vi "Board Power Control.vi"(8 "error in (no error)":errorcluster, 9 "VBUS":bool, 10 "Power-On":bool, 11 "CT Common Tests":refnum<class "CT Common Tests.lvclass">) -> (0 "error out":errorcluster, 3 "CT Common Tests":refnum<class "CT Common Tests.lvclass">)   [LabVIEW 2015, in "CT Common Tests.lvclass"]
uses:
  CT Common Tests.lvclass
  Classes/Instruments/Relay Control/Phidget Interface Kit/Class/Phidget Interface Kit 008.lvclass
  Classes/Application/Class/Application.lvclass
  Classes/Test Recipe/Class/Test Recipe.lvclass
  Test Class/Test Class.lvclass
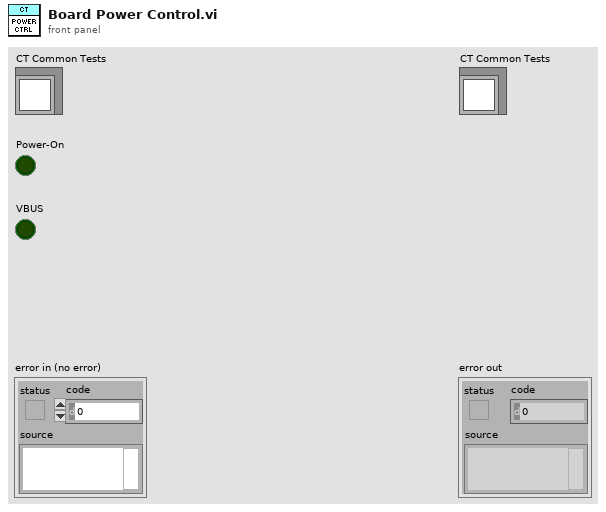
[diagram p1: front panel]
types:
  T1 = typedef "Application.lvlib/App Properties.lvclass/Class Properties -- Cluster.ctl" = cluster{"UUT Info":T2[], "Test Information":refnum<vi>, "Test Complete Event":refnum<user-event>, "Shop Floor System":refnum<class "Shop Floor System.lvclass">, "Gold Board":refnum<class "Golden Board.lvclass">, "Test Recipe":refnum<class "Test Recipe.lvclass">, "Instruments":refnum<class "Instrument.lvclass">[], "Mode":T3, "Test Results":cluster{"Pass":bool[], "Fail Codes":string[]}, "Station Config":refnum<class "Station Config.lvclass">}
  T2 = typedef "Application.lvlib/App Properties.lvclass/UUT Reference -- Cluster.ctl" = cluster{"Serial Number Reference":refnum<vi>, "Status Message Reference":refnum<vi>}
  T3 = typedef "Application.lvlib/Application.lvclass/Op Mode -- Enum.ctl" = u16
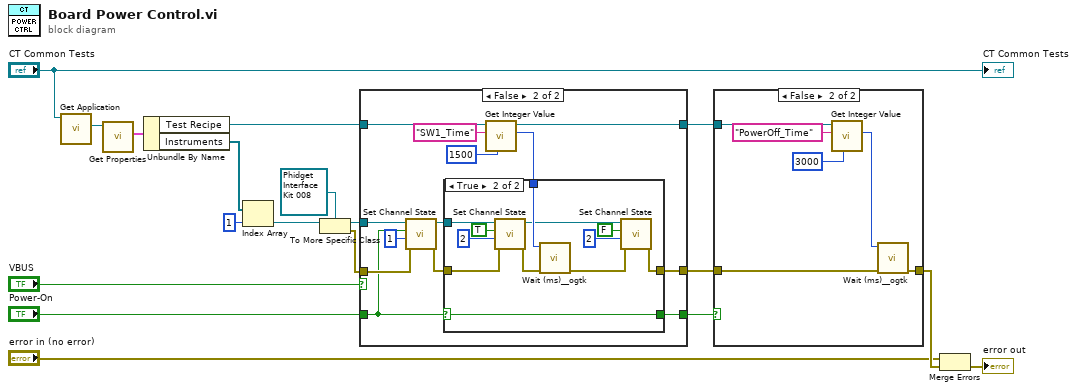
[diagram p0: block diagram]
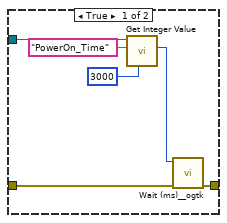
[diagram p2: hidden frame]
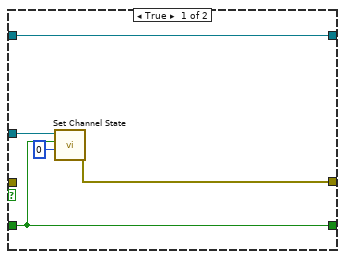
[diagram p3: hidden frame]
diagram:
  n1 = call "Get Application.vi"("Test Class in"="CT Common Tests") -> ("Application.lvlib:Application.lvclass"=w3:refnum<class "Application.lvclass">)  [unwired: 9 in, 1 out]
  n2 = call "Get Properties.vi"("Acrobat Template in"=w3) -> ("Class Properties"=w4:T1)  [unwired: 8 in, 2 out]
  n3 = Unbundle By Name(w4) -> ("Test Recipe"=w11:refnum<class "Test Recipe.lvclass">, "Instruments"=w5:refnum<class "Instrument.lvclass">[])
  n4 = Index Array(array=w5, index=1) -> (element=w7:refnum<class "Instrument.lvclass">)
  n5 = To More Specific Class(target class=refnum<class "Phidget Interface Kit 008.lvclass"> refnum ("Phidget Interface Kit 008.lvlib:Phidget Interface Kit 008.lvclass"), reference=w7) -> (specific class reference=w9:refnum<class "Phidget Interface Kit 008.lvclass">, error out=w13:errorcluster)  [unwired: 1 in]
  n6 = case shown="False" "VBUS" {
    tunnel: w9 -> [w22 w35]
    tunnel: "Power-On" -> [w19 w25]
    tunnel: [w21 w26] -> w10
    tunnel: w11 -> [w20 w32]
    tunnel: [w20 w31] -> w12
    tunnel: w13 -> [_ w28]
    tunnel: [w19 w24] -> w14
    frame True {
      n7 = call-dynamic "Set Channel State.vi"("Channel"=0, "State"=w19, "Acrobat Template in"=w22) -> ("error out"=w21:errorcluster)  [unwired: 7 in, 1 out]
    }
    frame False {
      n8 = call-dynamic "Set Channel State.vi"("error in (no error)"=w28, "Channel"=1, "State"=w25, "Acrobat Template in"=w35) -> ("error out"=w29:errorcluster, "Acrobat Template out"=w30:refnum<class "Phidget Interface Kit 008.lvclass">)  [unwired: 6 in]
      n9 = call "Get Integer Value.vi"("Default Value"=u32 1500, "Name"="SW1_Time", "Test Recipe in"=w32) -> ("Value"=w27:u32, "Test Recipe out"=w31:refnum<class "Test Recipe.lvclass">)  [unwired: 6 in, 1 out]
      n10 = case shown="True" w25 {
        selector: w25 -> [w37 w39]
        tunnel: w30 -> [_ w49]
        tunnel: w29 -> [w38 w47]
        tunnel: w27 -> [_ w46]
        tunnel: [w38 w42] -> w26
        tunnel: [w37 w39] -> w24
        frame False {
        }
        frame True {
          n11 = call-dynamic "Set Channel State.vi"("error in (no error)"=w47, "Channel"=2, "State"=TRUE, "Acrobat Template in"=w49) -> ("error out"=w45:errorcluster, "Acrobat Template out"=w41:refnum<class "Phidget Interface Kit 008.lvclass">)  [unwired: 6 in]
          n12 = call <userlib>:"Wait (ms)__ogtk.vi"("error in (no error)"=w45, "milliseconds to wait"=w46) -> ("error out"=w40:errorcluster)  [unwired: 8 in, 1 out]
          n13 = call-dynamic "Set Channel State.vi"("error in (no error)"=w40, "Channel"=2, "State"=FALSE, "Acrobat Template in"=w41) -> ("error out"=w42:errorcluster)  [unwired: 6 in, 1 out]
        }
      }
    }
  }
  n14 = case shown="False" w14 {
    tunnel: w10 -> [w54 w60]
    tunnel: [w52 w58] -> w18
    tunnel: w12 -> [w51 w57]
    frame True {
      n15 = call "Get Integer Value.vi"("Default Value"=u32 3000, "Name"="PowerOn_Time", "Test Recipe in"=w51) -> ("Value"=w53:u32)  [unwired: 6 in, 2 out]
      n16 = call <userlib>:"Wait (ms)__ogtk.vi"("error in (no error)"=w54, "milliseconds to wait"=w53) -> ("error out"=w52:errorcluster)  [unwired: 8 in, 1 out]
    }
    frame False {
      n17 = call "Get Integer Value.vi"("Default Value"=u32 3000, "Name"="PowerOff_Time", "Test Recipe in"=w57) -> ("Value"=w59:u32)  [unwired: 6 in, 2 out]
      n18 = call <userlib>:"Wait (ms)__ogtk.vi"("error in (no error)"=w60, "milliseconds to wait"=w59) -> ("error out"=w58:errorcluster)  [unwired: 8 in, 1 out]
    }
  }
  n19 = Merge Errors("error in (no error)", w18) -> (→"error out":errorcluster)
  "CT Common Tests" <- "CT Common Tests"
